vi "ResultView.vi"(8 "error in (no error)":errorcluster) -> (0 "error out":errorcluster)   [LabVIEW 2012]
uses:
  Signal/#TD_SignalStorageCommand.ctl
panel:
  in  "Stop Button":bool
  out "Waveform Graph":waveform(dbl)[](graph)
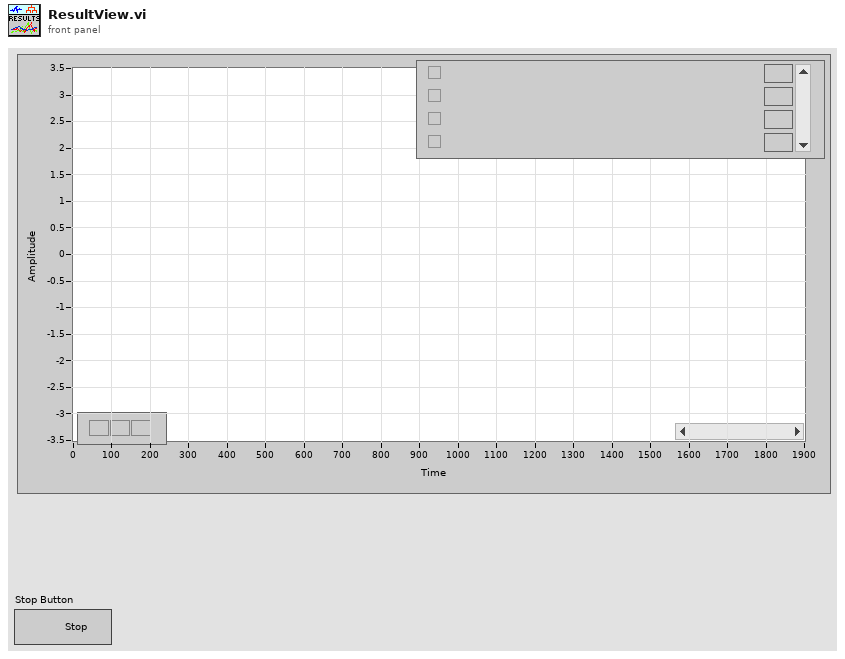
[diagram p1: front panel]
types:
  T1 = typedef "#TD_SignalStorageCommand.ctl" = enum16{"Reset_Storage", "Add_Signal", "Insert_Signal", "Del_Signal", "Replace_Signal", "Get_Signal", "Get_Signal_List", "Change_Signal_Name", "Change_Signal_Descr"}
  T2 = typedef "#TD_ThreadsStates.ctl" = cluster{"SigMgmntActive?":bool, "ResltVivActive?":bool, "SettngsMngActive?":bool}
  T3 = typedef "#TD_SignalStorageData.ctl" = cluster{"Signal Name":string, "Signal":waveform(dbl), "Description":string}
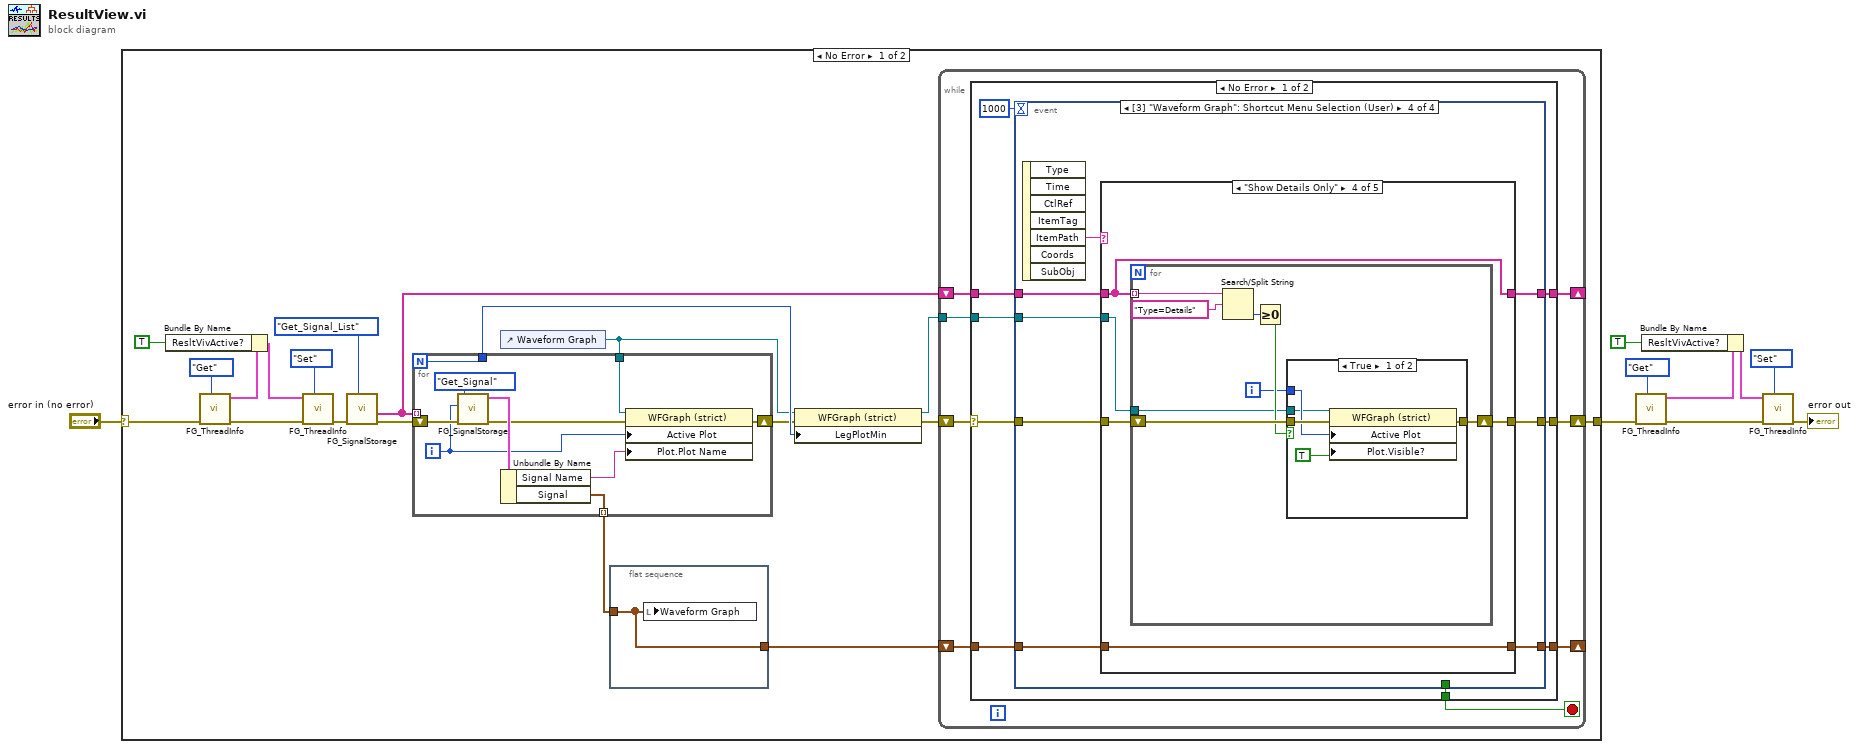
[diagram p0: block diagram]
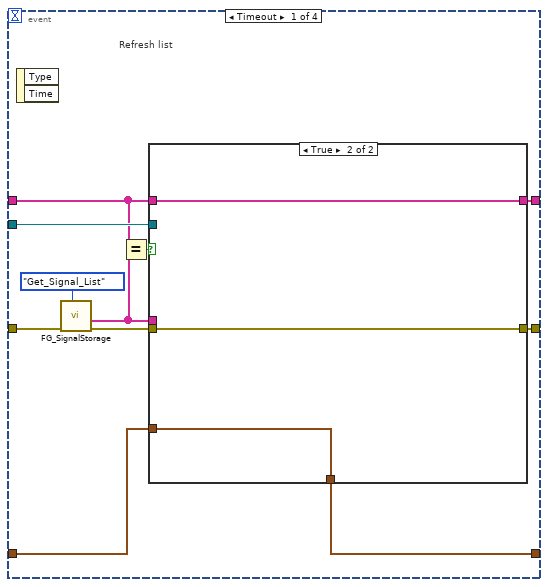
[diagram p2: hidden frame]
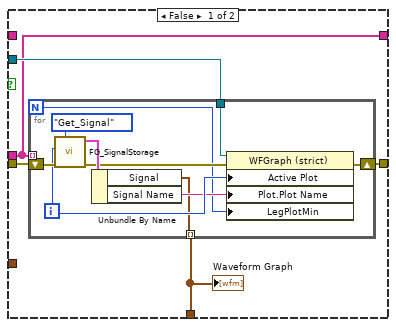
[diagram p3: hidden frame]
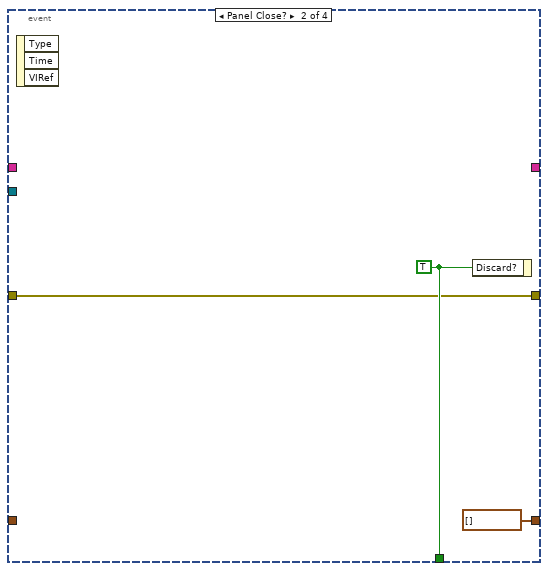
[diagram p4: hidden frame]
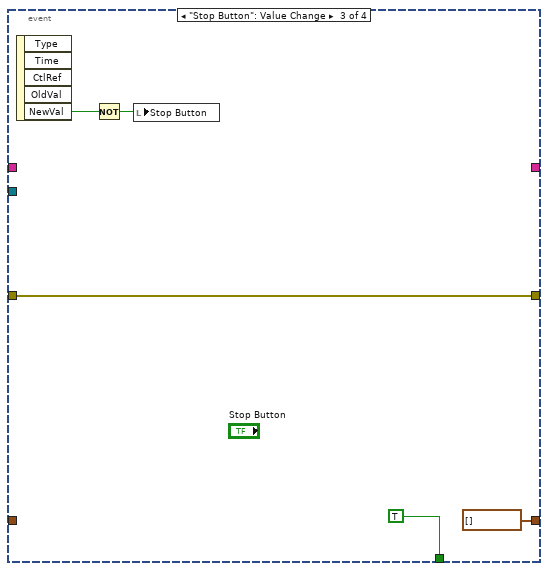
[diagram p5: hidden frame]
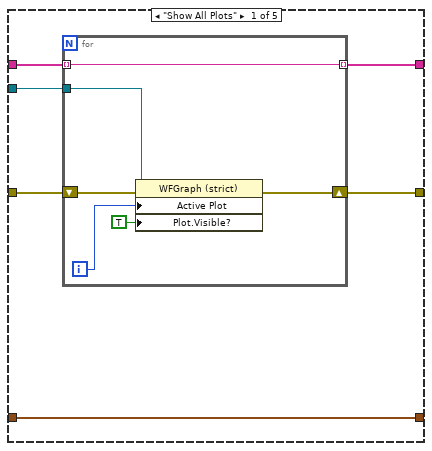
[diagram p6: hidden frame]
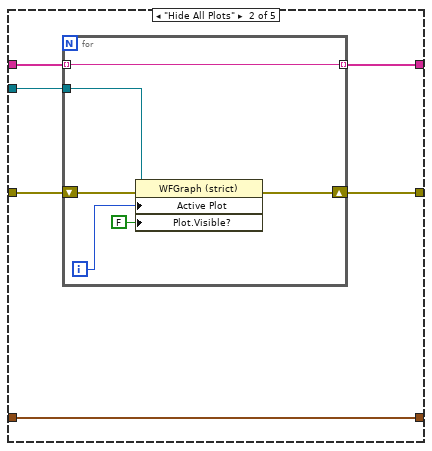
[diagram p7: hidden frame]
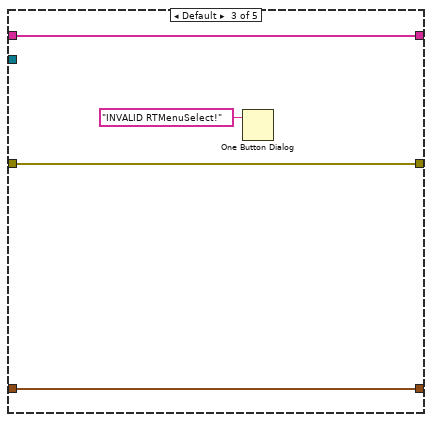
[diagram p8: hidden frame]
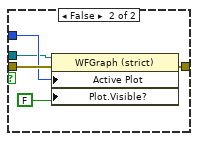
[diagram p9: hidden frame]
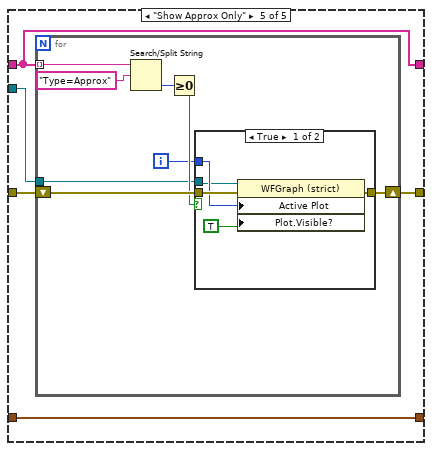
[diagram p10: hidden frame]
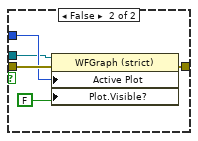
[diagram p11: hidden frame]
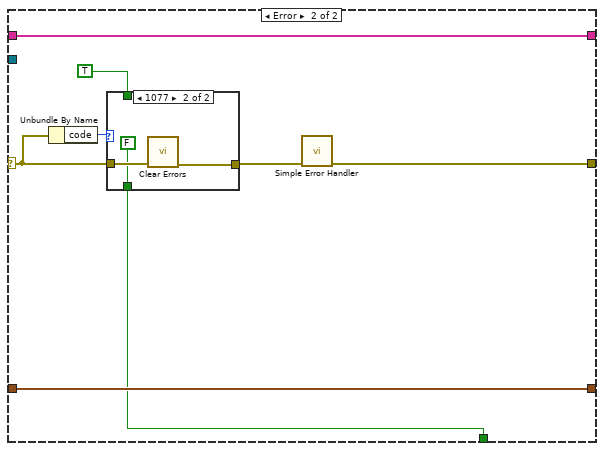
[diagram p12: hidden frame]
diagram:
  n1 = case shown="No Error" "error in (no error)" {
    selector: "error in (no error)" -> [w11 w189]
    tunnel: [w27 w189] -> w2
    frame No Error {
      n2 = call "FG_ThreadInfo.vi"("Command"=enum16{"Set", "Get"}."Get", "error in (no error)"=w11) -> ("error out"=w16:errorcluster, "ThreadsStates Out"=w14:T2)  [unwired: 8 in]
      n3 = Bundle By Name(cluster=w14, "ResltVivActive?"=TRUE ("SigMgmntActive?")) -> (w13:T2)
      n4 = call "FG_ThreadInfo.vi"("Command"=enum16{"Set", "Get"}."Set", "error in (no error)"=w16, "ThreadsStates"=w13) -> ("error out"=w10:errorcluster)  [unwired: 7 in, 1 out]
      n5 = call "FG_SignalStorage.vi"("Command"=#TD_SignalStorageCommand."Get_Signal_List", "error in (no error)"=w10) -> ("error out"=w25:errorcluster, "Signal_List"=w26:string[])  [unwired: 7 in, 1 out]
      n6 = control-ref of="Waveform Graph"() -> (w18:refnum<vi>)
      n7 = for {
        N -> [w32]
        tunnel: w26 -> [_] mode=indexing
        shift-right: [w35] -> w20
        shift-left: w25 -> [w39]
        tunnel: w18 -> [w33]
        tunnel: [w34] -> w24 mode=indexing
        tunnel: [w32] -> w21
        i -> [w30]
        n8 = call "FG_SignalStorage.vi"("Command"=#TD_SignalStorageCommand."Get_Signal", "error in (no error)"=w39, "SignalNumber"=w30) -> ("error out"=w36:errorcluster, "DataOut"=w37:T3)  [unwired: 6 in, 1 out]
        n9 = Unbundle By Name(w37) -> ("Signal Name"=w31:string, "Signal"=w34:waveform(dbl))
        n10 = property class="WFGraph (strict)"(reference=w33, error in=w36, "Active Plot"=w30, "Plot.Plot Name"=w31) -> (error out=w35:errorcluster)  [unwired: 1 out]
      }
      n11 = flat-sequence {
        tunnel: w24 -> [w29]
        tunnel: [w29] -> w23
        frame #0 {
          n12 = local write "Waveform Graph"(w29) -> ()
        }
      }
      n13 = property class="WFGraph (strict)"(reference=w18, error in=w20, "LegPlotMin"=w21) -> (reference out=w22:refnum<vi>, error out=w19:errorcluster)
      n14 = while {
        shift-right: [w46] -> w27
        shift-left: w19 -> [w44]
        shift-right: [w45] -> _
        shift-left: w23 -> [w43]
        tunnel: w22 -> [w42]
        shift-right: [w40] -> _
        shift-left: w26 -> [w41]
        stop <- w47 stop-if-true
        n15 = case shown="No Error" w44 {
          selector: w44 -> [w52 w179]
          tunnel: [w56 w177] -> w47
          tunnel: [w54 w181] -> w46
          tunnel: [w53 w182] -> w45
          tunnel: w43 -> [w51 w182]
          tunnel: w42 -> [w50 _]
          tunnel: w41 -> [w49 w183]
          tunnel: [w48 w183] -> w40
          frame No Error {
            n16 = event shown="[3] \"Waveform Graph\": Shortcut Menu Selection (User)" {
              selector: _ -> [_ _ _ _]
              dyn-events: _ -> [_ _ _ _]
              timeout: 1000 -> [_ _ _ _]
              tunnel: [_ w88 TRUE _] -> w56
              tunnel: w52 -> [w66 w87 w93 w99]
              tunnel: [w62 w87 w93 w100] -> w54
              tunnel: [w58 waveform(dbl)[] [] waveform(dbl)[] [] w98] -> w53
              tunnel: w51 -> [w59 _ _ w97]
              tunnel: w50 -> [w60 _ _ w94]
              tunnel: w49 -> [w57 _ _ w95]
              tunnel: [w61 _ _ w96] -> w48
              event Timeout {
                # "Refresh list"
                n17 = event-data() -> ()  [unwired: 1 in, 2 out]
                n18 = call "FG_SignalStorage.vi"("Command"=#TD_SignalStorageCommand."Get_Signal_List", "error in (no error)"=w66) -> ("error out"=w63:errorcluster, "Signal_List"=w64:string[])  [unwired: 7 in, 1 out]
                n19 = Equal?(x=w57, y=w64) -> (x = y?=w65:bool)
                n20 = case shown="True" w65 {
                  tunnel: w64 -> [w69 _]
                  tunnel: w63 -> [w70 w85]
                  tunnel: [w71 w85] -> w62
                  tunnel: [w69 w83] -> w61
                  tunnel: w59 -> [_ w84]
                  tunnel: w60 -> [w72 _]
                  tunnel: [w68 w84] -> w58
                  tunnel: w57 -> [_ w83]
                  frame False {
                    n21 = for {
                      N -> [w73]
                      shift-right: [w78] -> w71
                      shift-left: w70 -> [w82]
                      tunnel: w72 -> [w77]
                      tunnel: [w74] -> w68 mode=indexing
                      tunnel: w69 -> [_] mode=indexing
                      i -> [w76]
                      n22 = call "FG_SignalStorage.vi"("Command"=#TD_SignalStorageCommand."Get_Signal", "error in (no error)"=w82, "SignalNumber"=w76) -> ("error out"=w79:errorcluster, "DataOut"=w80:T3)  [unwired: 6 in, 1 out]
                      n23 = Unbundle By Name(w80) -> ("Signal"=w74:waveform(dbl), "Signal Name"=w75:string)
                      n24 = property class="WFGraph (strict)"(reference=w77, error in=w79, "Active Plot"=w76, "Plot.Plot Name"=w75, "LegPlotMin"=w73) -> (error out=w78:errorcluster)  [unwired: 1 out]
                    }
                    "Waveform Graph" <- w68
                  }
                  frame True {
                  }
                }
              }
              event Panel Close? {
                w88 = TRUE ("Discard?")
                n25 = event-data() -> ()  [unwired: 1 in, 3 out]
                n26 = event-data("Discard?"=w88) -> ()  [unwired: 1 in, 1 out]
              }
              event "Stop Button": Value Change {
                n27 = event-data() -> ("NewVal"=w90:bool)  [unwired: 1 in, 4 out]
                n28 = Not(x=w90) -> (.not. x?=w89:bool)
                n29 = local write "Stop Button"(w89) -> ()
              }
              event "Waveform Graph": Shortcut Menu Selection (User) {
                n30 = event-data() -> ("ItemPath"=w101:string)  [unwired: 1 in, 6 out]
                n31 = case shown="\"Show Details Only\"" w101 {
                  tunnel: [w103 w115 w129 w131 w154] -> w100
                  tunnel: w99 -> [w107 w119 w129 w132 w155]
                  tunnel: [w106 w118 w128 w134 w157] -> w98
                  tunnel: w97 -> [w106 w118 w128 w134 w157]
                  tunnel: [w102 w114 w127 w133 w156] -> w96
                  tunnel: w95 -> [w105 w117 w127 w133 w156]
                  tunnel: w94 -> [w104 w116 _ w130 w153]
                  frame "Show All Plots" {
                    n32 = for {
                      tunnel: w105 -> [w108] mode=indexing
                      tunnel: w104 -> [w111]
                      tunnel: [w108] -> w102 mode=indexing
                      shift-right: [w109] -> w103
                      shift-left: w107 -> [w113]
                      i -> [w112]
                      n33 = property class="WFGraph (strict)"(reference=w111, error in=w113, "Active Plot"=w112, "Plot.Visible?"=TRUE ("Plot.Visible")) -> (error out=w109:errorcluster)  [unwired: 1 out]
                    }
                  }
                  frame "Hide All Plots" {
                    n34 = for {
                      tunnel: w117 -> [w120] mode=indexing
                      tunnel: w116 -> [w123]
                      tunnel: [w120] -> w114 mode=indexing
                      shift-right: [w121] -> w115
                      shift-left: w119 -> [w125]
                      i -> [w124]
                      n35 = property class="WFGraph (strict)"(reference=w123, error in=w125, "Active Plot"=w124, "Plot.Visible?"=FALSE ("Plot.Visible")) -> (error out=w121:errorcluster)  [unwired: 1 out]
                    }
                  }
                  frame Default {
                    n36 = One Button Dialog(message="INVALID RTMenuSelect!") -> ()  [unwired: 1 in, 1 out]
                  }
                  frame "Show Details Only" {
                    n37 = for {
                      tunnel: w133 -> [w142] mode=indexing
                      shift-right: [w138] -> w131
                      shift-left: w132 -> [w139]
                      tunnel: w130 -> [w135]
                      i -> [w136]
                      n38 = Search/Split String(string=w142, search string/char (-)="Type=Details" ("regular expression")) -> (offset of match=w140:i32)  [unwired: 1 in, 2 out]
                      n39 = Greater Or Equal To 0?(x=w140) -> (x >= 0?=w137:bool)
                      n40 = case shown="True" w137 {
                        tunnel: w139 -> [w146 w151]
                        tunnel: [w145 w150] -> w138
                        tunnel: w136 -> [w144 w149]
                        tunnel: w135 -> [w143 w148]
                        frame True {
                          n41 = property class="WFGraph (strict)"(reference=w143, error in=w146, "Active Plot"=w144, "Plot.Visible?"=TRUE ("Plot.Visible")) -> (error out=w145:errorcluster)  [unwired: 1 out]
                        }
                        frame False {
                          n42 = property class="WFGraph (strict)"(reference=w148, error in=w151, "Active Plot"=w149, "Plot.Visible?"=FALSE ("Plot.Visible")) -> (error out=w150:errorcluster)  [unwired: 1 out]
                        }
                      }
                    }
                  }
                  frame "Show Approx Only" {
                    n43 = for {
                      tunnel: w156 -> [w165] mode=indexing
                      shift-right: [w161] -> w154
                      shift-left: w155 -> [w162]
                      tunnel: w153 -> [w158]
                      i -> [w159]
                      n44 = Search/Split String(string=w165, search string/char (-)="Type=Approx" ("regular expression")) -> (offset of match=w163:i32)  [unwired: 1 in, 2 out]
                      n45 = Greater Or Equal To 0?(x=w163) -> (x >= 0?=w160:bool)
                      n46 = case shown="True" w160 {
                        tunnel: w162 -> [w169 w174]
                        tunnel: [w168 w173] -> w161
                        tunnel: w159 -> [w167 w172]
                        tunnel: w158 -> [w166 w171]
                        frame True {
                          n47 = property class="WFGraph (strict)"(reference=w166, error in=w169, "Active Plot"=w167, "Plot.Visible?"=TRUE ("Plot.Visible")) -> (error out=w168:errorcluster)  [unwired: 1 out]
                        }
                        frame False {
                          n48 = property class="WFGraph (strict)"(reference=w171, error in=w174, "Active Plot"=w172, "Plot.Visible?"=FALSE ("Plot.Visible")) -> (error out=w173:errorcluster)  [unwired: 1 out]
                        }
                      }
                    }
                  }
                }
              }
            }
          }
          frame Error {
            n49 = Unbundle By Name(w179) -> ("code"=w180:i32)
            n50 = case shown="1077" w180 {
              tunnel: w179 -> [w185 w188]
              tunnel: [w185 w187] -> w178
              tunnel: [w184 FALSE] -> w177
              tunnel: TRUE -> [w184 _]
              frame 0, Default {
              }
              frame 1077 {
                n51 = call <vilib>:"Clear Errors.vi"("error in (no error)"=w188) -> ("error out"=w187:errorcluster)  [unwired: 6 in]
              }
            }
            n52 = call <vilib>:"Simple Error Handler.vi"("error in (no error)"=w178) -> ("error out"=w181:errorcluster)  [unwired: 4 in, 4 out]
          }
        }
      }
    }
    frame Error {
    }
  }
  n53 = call "FG_ThreadInfo.vi"("Command"=enum16{"Set", "Get"}."Get", "error in (no error)"=w2) -> ("error out"=w7:errorcluster, "ThreadsStates Out"=w5:T2)  [unwired: 8 in]
  n54 = Bundle By Name(cluster=w5, "ResltVivActive?"=TRUE ("SigMgmntActive?")) -> (w4:T2)
  n55 = call "FG_ThreadInfo.vi"("Command"=enum16{"Set", "Get"}."Set", "error in (no error)"=w7, "ThreadsStates"=w4) -> ("error out"=→"error out":errorcluster)  [unwired: 7 in, 1 out]
